vi "Read DetailedResult.vi"(8 "error in (no error)":errorcluster, 11 "TestDetailedResult in":refnum<class "TestDetailedResult.lvclass">) -> (0 "error out":errorcluster, 2 "DetailedResult":T1, 3 "TestDetailedResult out":refnum<class "TestDetailedResult.lvclass">)   [LabVIEW 2019, in "TestEngine.lvlib" / "TestDetailedResult.lvclass"]
uses:
  TestDetailedResult.lvclass
  TestDetailedResult.lvclass/TestDetailedResult.ctl
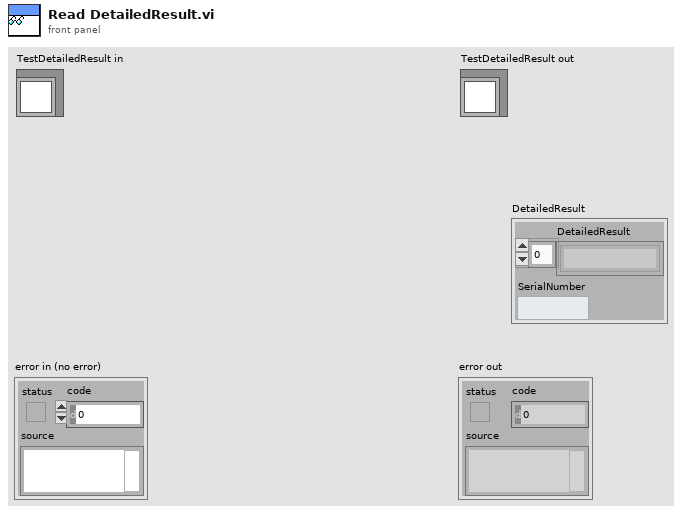
[diagram p1: front panel]
types:
  T1 = cluster{"DetailedResult":string[], "SerialNumber":string}
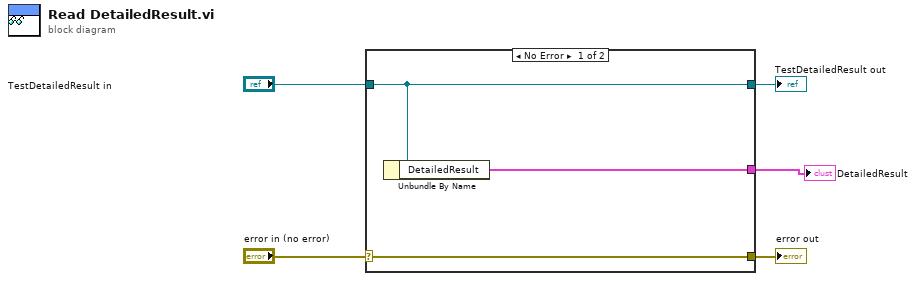
[diagram p0: block diagram]
diagram:
  n1 = case shown="No Error" "error in (no error)" {
    selector: "error in (no error)" -> [w8 w9]
    tunnel: [w8 w9] -> w4
    tunnel: [w7 w10] -> w2
    tunnel: "TestDetailedResult in" -> [w7 w10]
    tunnel: [w6 _] -> w1
    frame No Error {
      n2 = Unbundle By Name(w7) -> ("DetailedResult"=w6:T1)
    }
    frame Error {
    }
  }
  "error out" <- w4
  "TestDetailedResult out" <- w2
  "DetailedResult" <- w1
